vi "FromJason.vi"(8 "error in (no error)":errorcluster, 10 "String":string) -> (0 "error out":errorcluster, 3 "Flags out":refnum<class "Flags.lvclass">)   [LabVIEW 2015, in "Flags.lvclass"]
uses:
  Flags.lvclass
  JasonCluster.ctl
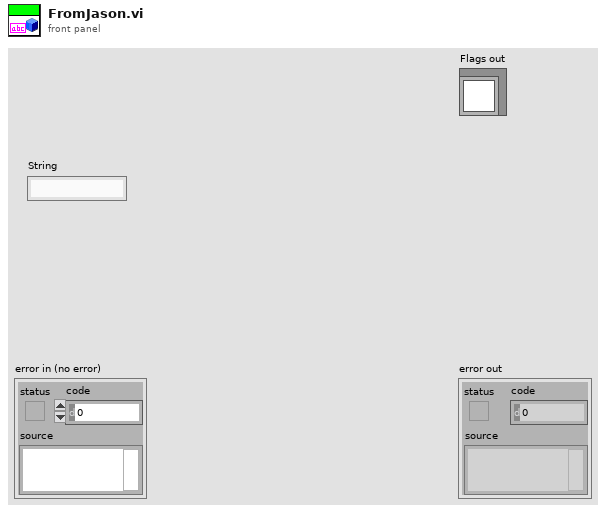
[diagram p1: front panel]
types:
  T1 = typedef "Flags.lvclass/JasonCluster.ctl" = cluster{"State":bool[], "Color":i32[], "Room Number":u32}
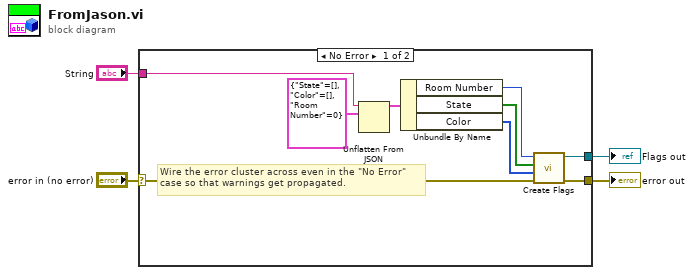
[diagram p0: block diagram]
diagram:
  n1 = case shown="No Error" "error in (no error)" {
    selector: "error in (no error)" -> [w7 w14]
    tunnel: [w6 w14] -> w3
    tunnel: [w5 _] -> w2
    tunnel: "String" -> [w13 _]
    frame No Error {
      # "Wire the error cluster across even in the \"No Error\"\ncase so that warnings get propagated."
      n2 = Unflatten From JSON(JSON string=w13, type and defaults=T1 {"State"=[], "Color"=[], "Room Number"=0} ("Cluster of class private data")) -> (value=w11:T1)  [unwired: 5 in, 1 out]
      n3 = Unbundle By Name(w11) -> ("Room Number"=w10:u32, "State"=w9:bool[], "Color"=w8:i32[])
      n4 = call "Create Flags.vi"("error in"=w7, "Color"=w8, "State"=w9, "Room Number"=w10) -> ("error out"=w6:errorcluster, "reference out"=w5:refnum<class "Flags.lvclass">)  [unwired: 6 in]
    }
    frame Error {
    }
  }
  "error out" <- w3
  "Flags out" <- w2
